vi "dump_name.vi"(11 "section/key":string[](array[string])) -> (3 "toml":string)   [LabVIEW 2017, in "rpacini_toml.lvlib"]
uses:
  rpacini_toml.lvlib
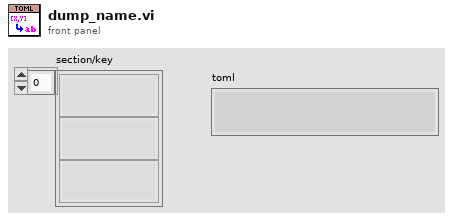
[diagram p1: front panel]
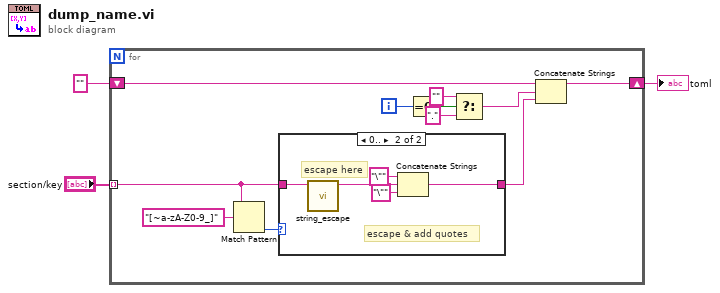
[diagram p0: block diagram]
diagram:
  n1 = for {
    tunnel: "section/key" -> [w12] mode=indexing
    shift-right: [w10] -> w1
    shift-left: "" -> [w11]
    i -> [w8]
    n2 = Match Pattern(string=w12, regular expression="[~a-zA-Z0-9_]") -> (offset past match=w13:i32)  [unwired: 1 in, 3 out]
    n3 = case shown="0.." w13 {
      tunnel: w12 -> [w15 w17]
      tunnel: [w15 w20] -> w9
      frame ..-1 {
      }
      frame 0.. {
        # "escape here"
        # "escape & add quotes"
        n4 = call "string_escape.vi"("string"=w17) -> ("escaped string"=w16:string)  [unwired: 10 in]
        n5 = Concatenate Strings("\"" ("string"), w16, "\"" ("string")) -> (w20:string)
      }
    }
    n6 = Equal To 0?(x=w8) -> (x = 0?=w7:bool)
    n7 = Select(t="", s=w7, f=".") -> (s? t:f=w4:string)
    n8 = Concatenate Strings(w11, w4, w9) -> (w10:string)
  }
  "toml" <- w1
